vi "Creators Is Created Event.vi"(10 "Created Event Alias":string, 11 "eeeee in":refnum<class "eeeee.lvclass">) -> (2 "Is Created Event?":bool, 3 "eeeee out":refnum<class "eeeee.lvclass">)   [LabVIEW 2021, in "jettl Tools.lvlib" / "eeeee.lvlib" / "eeeee.lvclass"]
uses:
  eeeee.lvclass
  eeeee.lvclass/eeeee.ctl
  jettl/Event/Event.lvclass
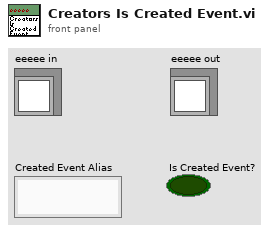
[diagram p1: front panel]
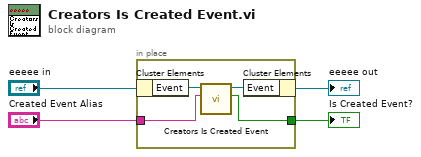
[diagram p0: block diagram]
diagram:
  n1 = in-place {
    in-place-border: [w6] -> w2
    in-place-border: "Created Event Alias" -> [w5]
    n2 = in-place-cluster #1("eeeee in") -> ("Event"=w8:refnum<class "Event.lvclass">)
    n3 = call-dynamic "Creators Is Created Event.vi"("Created Event Alias"=w5, "Event in"=w8) -> ("Is Created Event?"=w6:bool, "Event out"=w7:refnum<class "Event.lvclass">)  [unwired: 8 in]
    n4 = in-place-cluster #1("Event"=w7) -> (→"eeeee out":refnum<class "eeeee.lvclass">)
  }
  "Is Created Event?" <- w2
